vi "Main.vi"() -> ()   [LabVIEW 2020, in "Signal Generator App.lvclass"]
uses:
  Signal Generator App.lvclass
  Composite Waveform/Composite Waveform.lvclass
  C:/Users/fflores/Documents/GitHub Projects/OOP-Concepts-in-LabVIEW/Design Patterns/Composite Pattern/Analog Waveform/Analog Waveform.lvclass
  Analog Waveform/Analog Waveform.lvclass
  Sine/Sine.lvclass
  Tirangle/Tirangle.lvclass
panel:
  in  "index":i32
  in  "Add Button":bool
  out "Composite waveform":waveform(dbl)(graph)
  out "Waveform Graph":waveform(dbl)(graph)
  in  "Phase":dbl(knob) step=0.1 scale=0.0..360.0
  in  "Offset":dbl(knob) step=0.1 scale=-10.0..10.0
  in  "Frequency":dbl(knob) step=0.1 scale=0.0..10.0
  in  "Amplitude":dbl(knob) step=0.1 scale=0.0..10.0
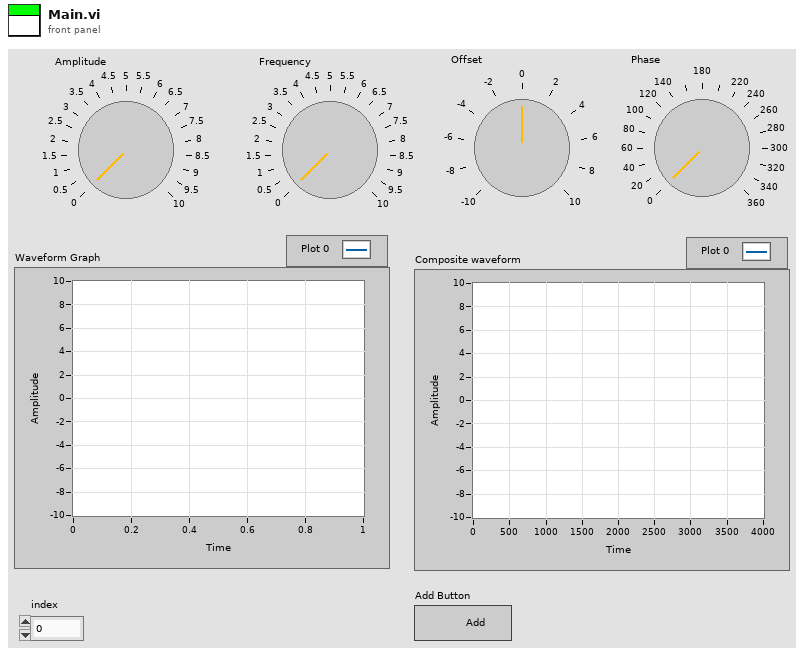
[diagram p1: front panel]
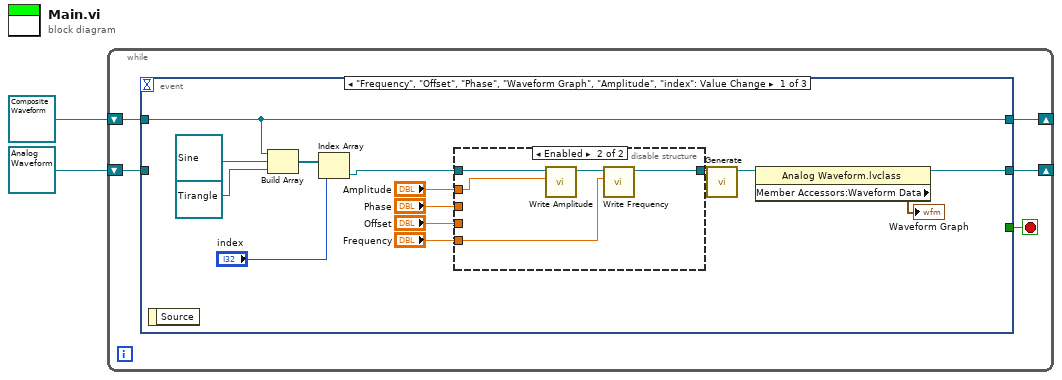
[diagram p0: block diagram]
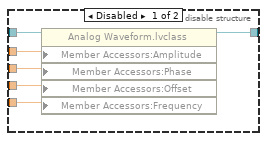
[diagram p2: hidden frame]
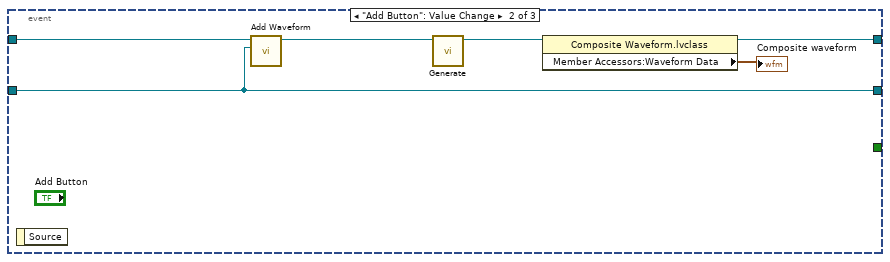
[diagram p3: hidden frame]
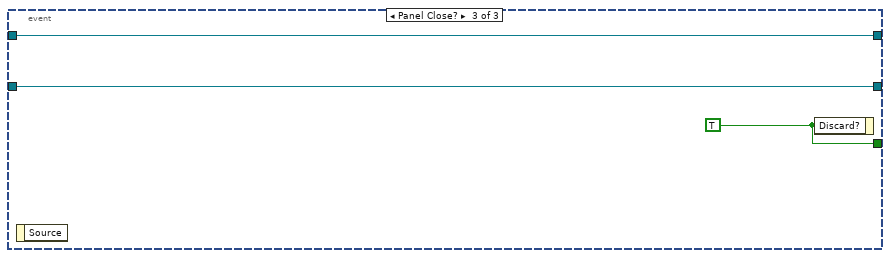
[diagram p4: hidden frame]
diagram:
  n1 = while {
    shift-right: [w6] -> _
    shift-left: refnum<class "Analog Waveform.lvclass"> refnum ("Analog Waveform.lvclass") -> [w7]
    shift-right: [w3] -> _
    shift-left: refnum<class "Composite Waveform.lvclass"> refnum ("Composite Waveform.lvclass") -> [w4]
    stop <- w5 stop-if-true
    n2 = event shown="[0] \"Frequency\", \"Offset\", \"Phase\", \"Waveform Graph\", \"Amplitude\", \"index\": Value Change" {
      selector: _ -> [_ _ _]
      dyn-events: _ -> [_ _ _]
      timeout: _ -> [_ _ _]
      tunnel: w7 -> [_ w36 w41]
      tunnel: [w15 w36 w41] -> w6
      tunnel: [_ _ w40] -> w5
      tunnel: w4 -> [w13 w38 w39]
      tunnel: [w13 w34 w39] -> w3
      event "Frequency", "Offset", "Phase", "Waveform Graph", "Amplitude", "index": Value Change {
        n3 = event-data() -> ()  [unwired: 1 in, 1 out]
        n4 = Build Array(w13, refnum<class "Sine.lvclass"> refnum ("Sine.lvclass"), refnum<class "Tirangle.lvclass"> refnum ("Tirangle.lvclass")) -> (w10:refnum<class "Analog Waveform.lvclass">[])
        n5 = Index Array(array=w10, index="index") -> (element=w9:refnum<class "Analog Waveform.lvclass">)
        n6 = disable-structure shown="Enabled" {
          disable-tunnel: [w27 w29] -> w21
          disable-tunnel: "Amplitude" -> [w26 w30]
          disable-tunnel: "Phase" -> [w25 _]
          disable-tunnel: "Offset" -> [w24 _]
          disable-tunnel: "Frequency" -> [w23 w28]
          disable-tunnel: w9 -> [w22 w32]
          frame Disabled {
            n7 = property class="Analog Waveform.lvclass"(reference=w22, "Member Accessors:Amplitude"=w26, "Member Accessors:Phase"=w25, "Member Accessors:Offset"=w24, "Member Accessors:Frequency"=w23) -> (reference out=w27:refnum<class "Analog Waveform.lvclass">)  [unwired: 1 in, 1 out]
          }
          frame Enabled {
            n8 = call-dynamic "Write Amplitude.vi"("Amplitude"=w30, "Analog Waveform in"=w32) -> ("Analog Waveform out"=w31:refnum<class "Analog Waveform.lvclass">)  [unwired: 8 in, 1 out]
            n9 = call-dynamic "Write Frequency.vi"("Frequency"=w28, "Analog Waveform in"=w31) -> ("Analog Waveform out"=w29:refnum<class "Analog Waveform.lvclass">)  [unwired: 8 in, 1 out]
          }
        }
        n10 = call-dynamic "Generate.vi"("Analog Waveform in"=w21) -> ("Analog Waveform out"=w16:refnum<class "Analog Waveform.lvclass">)  [unwired: 9 in, 1 out]
        n11 = property class="Analog Waveform.lvclass"(reference=w16) -> (reference out=w15:refnum<class "Analog Waveform.lvclass">, "Member Accessors:Waveform Data"=→"Waveform Graph":waveform(dbl))  [unwired: 1 in, 1 out]
      }
      event "Add Button": Value Change {
        n12 = event-data() -> ()  [unwired: 1 in, 1 out]
        n13 = call "Add Waveform.vi"("Waveform"=w36, "Composite Waveform in"=w38) -> ("Composite Waveform out"=w37:refnum<class "Composite Waveform.lvclass">)  [unwired: 8 in, 1 out]
        n14 = call-dynamic "Generate.vi"("Composite Waveform in"=w37) -> ("Composite Waveform out"=w35:refnum<class "Composite Waveform.lvclass">)  [unwired: 9 in, 1 out]
        n15 = property class="Composite Waveform.lvclass"(reference=w35) -> (reference out=w34:refnum<class "Composite Waveform.lvclass">, "Member Accessors:Waveform Data"=→"Composite waveform":waveform(dbl))  [unwired: 1 in, 1 out]
      }
      event Panel Close? {
        w40 = TRUE ("Discard?")
        n16 = event-data() -> ()  [unwired: 1 in, 1 out]
        n17 = event-data("Discard?"=w40) -> ()  [unwired: 1 in, 1 out]
      }
    }
  }
